vi "K2400readconvert.vi"(11 "String":string="+5.028856E-02,+1.000011E-04,+9.910000E+37,+1.058732E+03,+3.994000E+04") -> (2 "current":dbl, 3 "voltage":dbl)   [LabVIEW 2019]
panel:
  out "Array":dbl[](array[numeric])
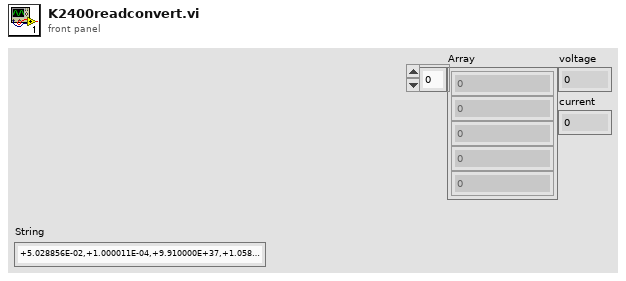
[diagram p1: front panel]
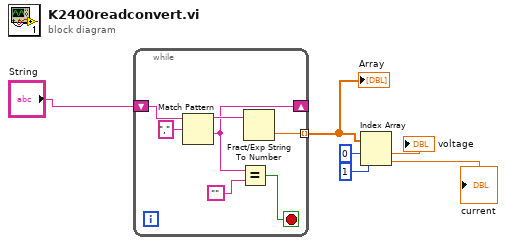
[diagram p0: block diagram]
diagram:
  n1 = while {
    tunnel: [w11] -> w5 mode=indexing
    shift-right: [w9] -> _
    shift-left: "String" -> [w10]
    stop <- w7 stop-if-true
    n2 = Match Pattern(string=w10, regular expression=",") -> (before substring=w12:string, after substring=w9:string)  [unwired: 1 in, 2 out]
    n3 = Equal?(x=w9, y="") -> (x = y?=w7:bool)
    n4 = Fract/Exp String To Number(string=w12) -> (number=w11:dbl)  [unwired: 3 in, 1 out]
  }
  "Array" <- w5
  n5 = Index Array(array=w5, index #1=0 ("index"), index #2=1 ("index")) -> (element #1=→"voltage":dbl, element #2=→"current":dbl)
